vi "系统执行module1文件.vi"() -> ()   [LabVIEW 2018]
panel:
  in  "working directory":path=path "C:/Users/86136/source/repos" caption="工作目录"
  in  "command line":string="python module1.py" caption="命令行"
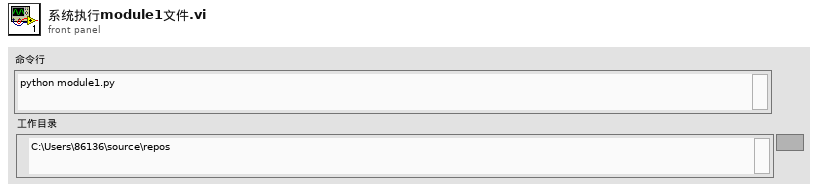
[diagram p1: front panel]
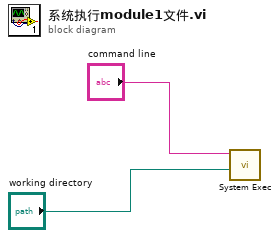
[diagram p0: block diagram]
diagram:
  n1 = call <vilib>:"System Exec.vi"("working directory"="working directory", "command line"="command line") -> ()  [unwired: 6 in, 4 out]
